vi "W9EO82,FBO8PP_6.vi"() -> ()   [LabVIEW 2021]
uses:
  <vilib>/measure/NI_MABase.lvlib
panel:
  out "Teljesítmény":dbl
  out "Waveform Graph 2":waveform(dbl)(graph)
  in  "duty cycle (%)":dbl=50.0 format="%0.2f"
  out "V effektiv":dbl
  out "Integral":dbl
  out "Waveform Graph":waveform(dbl)(graph)
  in  "offset":dbl format="%0.2p"
  in  "amplitudo":dbl=1.0 format="%0.2p"
  in  "frekvencia":dbl=10.0 format="%0.2p"
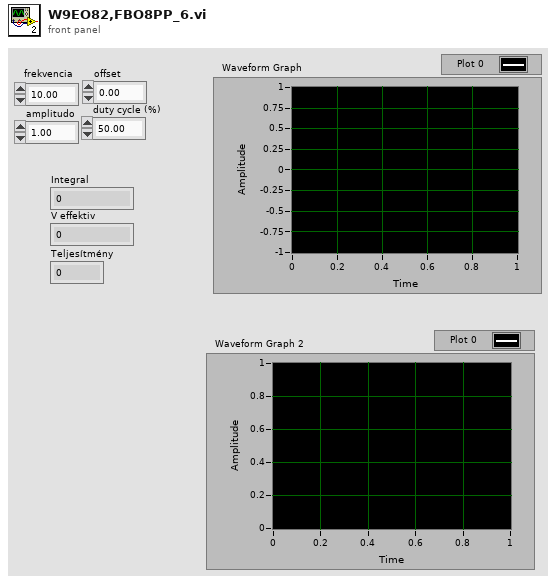
[diagram p1: front panel]
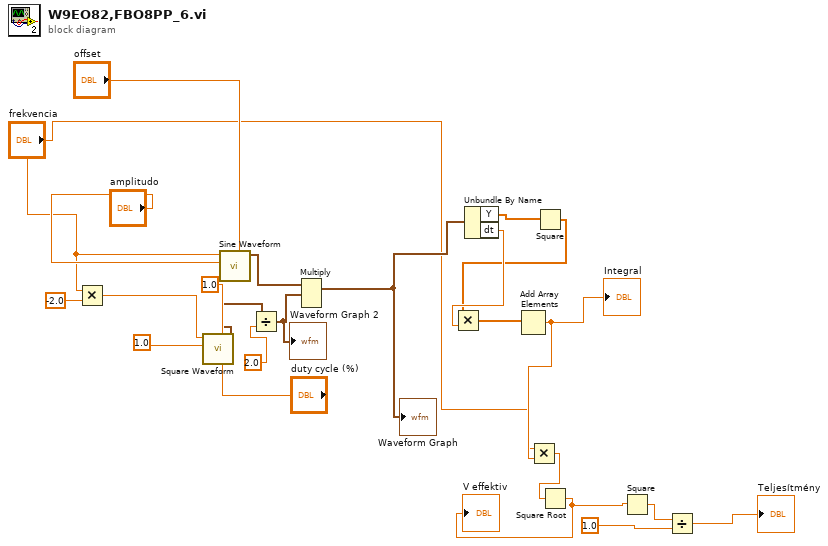
[diagram p0: block diagram]
diagram:
  n1 = Multiply(x="frekvencia", y=-2.0) -> (x*y=w5:dbl)
  n2 = call <vilib>:"Square Waveform.vi"("duty cycle (%)"="duty cycle (%)", "offset"=1.0, "amplitude"=1.0, "frequency"=w5) -> ("signal out"=w8:waveform(dbl))  [unwired: 6 in, 1 out]
  n3 = call <vilib>:"Sine Waveform.vi"("offset"="offset", "amplitude"="amplitudo", "frequency"="frekvencia") -> ("signal out"=w15:waveform(dbl))  [unwired: 7 in, 1 out]
  n4 = Divide(x=w8, y=2.0 ("x")) -> (x/y=w10:waveform(dbl))
  "Waveform Graph 2" <- w10
  n5 = Multiply(1:w10, 2:w15) -> (0:w14:waveform(dbl))  [unwired: 1 in, 1 out]
  "Waveform Graph" <- w14
  n6 = Unbundle By Name(w14) -> ("Y"=w18:dbl[], "dt"=w21:dbl)
  n7 = Square(x=w18) -> (x^2=w17:dbl[])
  n8 = Multiply(x=w17, y=w21) -> (x*y=w16:dbl[])
  n9 = Add Array Elements(numeric array=w16) -> (sum=w19:dbl)
  "Integral" <- w19
  n10 = Multiply(x="frekvencia", y=w19) -> (x*y=w20:dbl)
  n11 = Square Root(x=w20) -> (sqrt(x)=w2:dbl)
  "V effektiv" <- w2
  n12 = Square(x=w2) -> (x^2=w3:dbl)
  n13 = Divide(x=w3, y=1.0) -> (x/y=→"Teljesítmény":dbl)
